vi "Word_Format_Table_Range.vi"(4 "end column":i32, 5 "start column":i32, 6 "end row":i32, 7 "start row":i32, 8 "error in":errorcluster, 9 "font":T1 {"font size" format="%.2f"; "strike through" items=["Unchanged", "Yes", "No"]; "underline" items=["Unchanged", "Yes", "No"]; "italic" items=["Unchanged", "Yes", "No"]; "bold" items=["Unchanged", "Yes", "No"]}, 10 "table":refnum<k7>, 11 "Word._Application":refnum<k7>) -> (0 "error out":errorcluster)   [LabVIEW 2020, in "NI_ReportGenerationToolkit.lvlib"]
uses:
  <vilib>/addons/_office/NI_ReportGenerationToolkit.lvlib
  <vilib>/addons/_office/_exclsub.llb/font.ctl
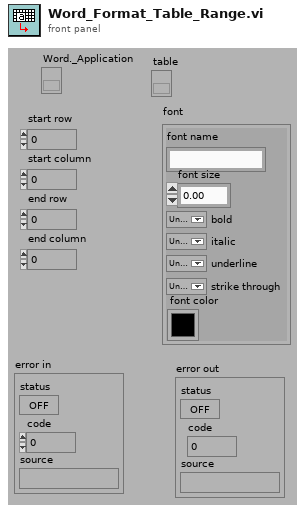
[diagram p1: front panel]
types:
  T1 = typedef "NI_ReportGenerationToolkit.lvlib/font.ctl" = cluster{"font name":string, "font size":dbl, "bold":u16, "italic":u16, "underline":u16, "strike through":u16, "font color":u32}
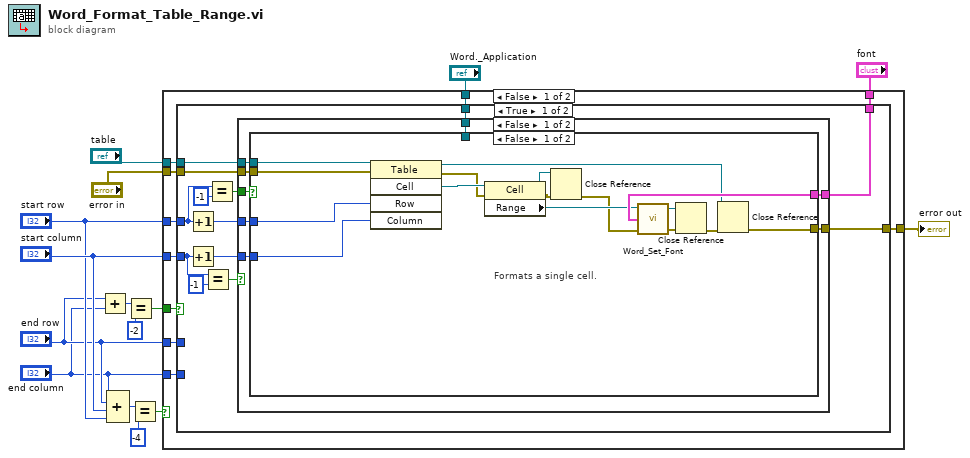
[diagram p0: block diagram]
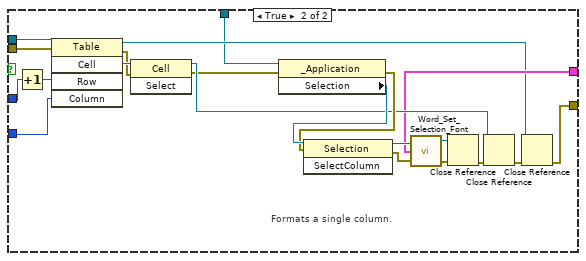
[diagram p2: hidden frame]
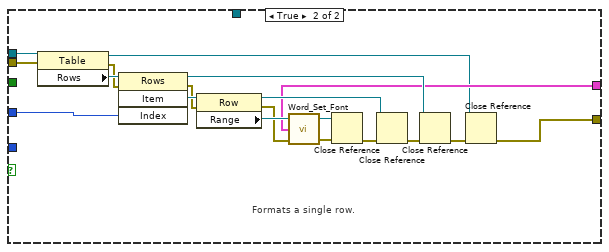
[diagram p3: hidden frame]
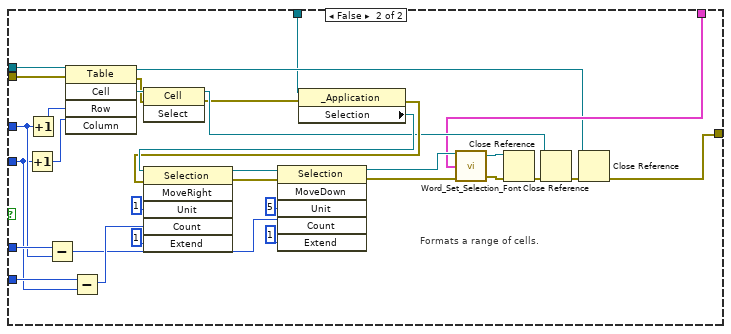
[diagram p4: hidden frame]
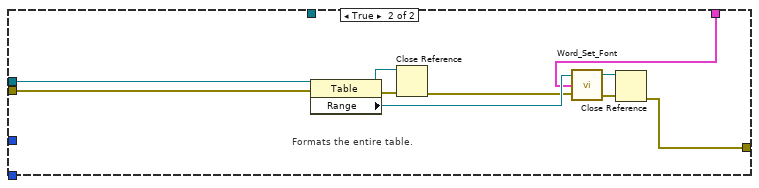
[diagram p5: hidden frame]
diagram:
  n1 = Add(x="end row", y="end column") -> (x+y=w6:i32)
  n2 = Compound Arithmetic op=ADD("end column", "end row", "start column", "start row") -> (w13:i32)
  n3 = Equal?(x=w6, y=-2) -> (x = y?=w4:bool)
  n4 = Equal?(x=w13, y=-4) -> (x = y?=w11:bool)
  n5 = case shown="False" w11 {
    tunnel: "start column" -> [w25 _]
    tunnel: "start row" -> [w24 _]
    tunnel: "end row" -> [w23 _]
    tunnel: "end column" -> [w22 _]
    tunnel: [w21 w138] -> w3
    tunnel: "table" -> [w20 w144]
    tunnel: "error in" -> [w19 w143]
    tunnel: w4 -> [w18 _]
    tunnel: "font" -> [w17 w141]
    tunnel: "Word._Application" -> [w16 _]
    frame False {
      n6 = case shown="True" w18 {
        tunnel: w25 -> [w31 w117]
        tunnel: w24 -> [w28 w118]
        tunnel: w23 -> [_ w120]
        tunnel: w22 -> [_ w119]
        tunnel: [w38 w107] -> w21
        tunnel: w20 -> [w36 w134]
        tunnel: w19 -> [w33 w133]
        tunnel: w17 -> [w37 w106]
        tunnel: w16 -> [w26 w103]
        frame True {
          n7 = Increment(x=w28) -> (x+1=w35:i32)
          n8 = Increment(x=w31) -> (x+1=w34:i32)
          n9 = Equal?(x=w31, y=-1) -> (x = y?=w32:bool)
          n10 = Equal?(x=w28, y=-1) -> (x = y?=w27:bool)
          n11 = case shown="False" w32 {
            tunnel: [w46 w85] -> w38
            tunnel: w37 -> [w45 w87]
            tunnel: w36 -> [w44 w102]
            tunnel: w35 -> [w43 w100]
            tunnel: w34 -> [w42 _]
            tunnel: w33 -> [w41 w92]
            tunnel: w27 -> [w40 _]
            tunnel: w26 -> [w39 _]
            frame False {
              n12 = case shown="False" w40 {
                tunnel: [w48 w72] -> w46
                tunnel: w45 -> [w58 w67]
                tunnel: w44 -> [w57 w81]
                tunnel: w43 -> [w56 w79]
                tunnel: w42 -> [w55 w78]
                tunnel: w41 -> [w53 w80]
                tunnel: w39 -> [_ w63]
                frame False {
                  # "Formats a single cell."
                  n13 = invoke class="Table" method="Cell"(reference=w57, error in=w53, "Row"=w56, "Column"=w55) -> (reference out=w47:refnum<k7>, error out=w52:errorcluster, "Cell"=w54:refnum<k7>)  [unwired: 1 in, 2 out]
                  n14 = property class="Cell"(reference=w54, error in=w52) -> (reference out=w62:refnum<k7>, error out=w61:errorcluster, "Range"=w51:refnum<k7>)
                  n15 = Close Reference(reference=w62, error in (no error)=w61) -> (error out=w50:errorcluster)
                  n16 = call <vilib>:"Word_Set_Font.vi"("Range in"=w51, "font"=w58, "Error in"=w50) -> ("Range out"=w59:refnum<k7>, "Error out"=w60:errorcluster)  [unwired: 5 out]
                  n17 = Close Reference(reference=w59, error in (no error)=w60) -> (error out=w49:errorcluster)
                  n18 = Close Reference(reference=w47, error in (no error)=w49) -> (error out=w48:errorcluster)
                }
                frame True {
                  # "Formats a single column."
                  n19 = Increment(x=w79) -> (x+1=w66:i32)
                  n20 = invoke class="Table" method="Cell"(reference=w81, error in=w80, "Row"=w66, "Column"=w78) -> (reference out=w65:refnum<k7>, error out=w76:errorcluster, "Cell"=w77:refnum<k7>)  [unwired: 1 in, 2 out]
                  n21 = invoke class="Cell" method="Select"(reference=w77, error in=w76) -> (reference out=w68:refnum<k7>, error out=w64:errorcluster)  [unwired: 1 in, 1 out]
                  n22 = property class="_Application"(reference=w63, error in=w64) -> (error out=w70:errorcluster, "Selection"=w71:refnum<k7>)  [unwired: 1 out]
                  n23 = invoke class="Selection" method="SelectColumn"(reference=w71, error in=w70) -> (reference out=w74:refnum<k7>, error out=w69:errorcluster)  [unwired: 1 in, 1 out]
                  n24 = call <vilib>:"Word_Set_Selection_Font.vi"("selection in"=w74, "font"=w67, "error in"=w69) -> ("selection out"=w75:refnum<k7>, "error out"=w83:errorcluster)  [unwired: 5 out]
                  n25 = Close Reference(reference=w75, error in (no error)=w83) -> (error out=w82:errorcluster)
                  n26 = Close Reference(reference=w68, error in (no error)=w82) -> (error out=w73:errorcluster)
                  n27 = Close Reference(reference=w65, error in (no error)=w73) -> (error out=w72:errorcluster)
                }
              }
            }
            frame True {
              # "Formats a single row."
              n28 = property class="Table"(reference=w102, error in=w92) -> (reference out=w84:refnum<k7>, error out=w95:errorcluster, "Rows"=w101:refnum<k7>)
              n29 = invoke class="Rows" method="Item"(reference=w101, error in=w95, "Index"=w100) -> (reference out=w88:refnum<k7>, error out=w94:errorcluster, "Item"=w99:refnum<k7>)  [unwired: 1 in, 1 out]
              n30 = property class="Row"(reference=w99, error in=w94) -> (reference out=w89:refnum<k7>, error out=w93:errorcluster, "Range"=w96:refnum<k7>)
              n31 = call <vilib>:"Word_Set_Font.vi"("Range in"=w96, "font"=w87, "Error in"=w93) -> ("Range out"=w97:refnum<k7>, "Error out"=w98:errorcluster)  [unwired: 5 out]
              n32 = Close Reference(reference=w97, error in (no error)=w98) -> (error out=w91:errorcluster)
              n33 = Close Reference(reference=w89, error in (no error)=w91) -> (error out=w90:errorcluster)
              n34 = Close Reference(reference=w88, error in (no error)=w90) -> (error out=w86:errorcluster)
              n35 = Close Reference(reference=w84, error in (no error)=w86) -> (error out=w85:errorcluster)
            }
          }
        }
        frame False {
          # "Formats a range of cells."
          n36 = Increment(x=w117) -> (x+1=w131:i32)
          n37 = Increment(x=w118) -> (x+1=w132:i32)
          n38 = Subtract(x=w120, y=w118) -> (x-y=w115:i32)
          n39 = invoke class="Table" method="Cell"(reference=w134, error in=w133, "Row"=w132, "Column"=w131) -> (reference out=w105:refnum<k7>, error out=w129:errorcluster, "Cell"=w130:refnum<k7>)  [unwired: 1 in, 2 out]
          n40 = Subtract(x=w119, y=w117) -> (x-y=w116:i32)
          n41 = invoke class="Cell" method="Select"(reference=w130, error in=w129) -> (reference out=w108:refnum<k7>, error out=w104:errorcluster)  [unwired: 1 in, 1 out]
          n42 = property class="_Application"(reference=w103, error in=w104) -> (error out=w127:errorcluster, "Selection"=w128:refnum<k7>)  [unwired: 1 out]
          n43 = invoke class="Selection" method="MoveRight"(reference=w128, error in=w127, "Unit"=1, "Count"=w116, "Extend"=1) -> (reference out=w124:refnum<k7>, error out=w123:errorcluster)  [unwired: 1 in, 4 out]
          n44 = invoke class="Selection" method="MoveDown"(reference=w124, error in=w123, "Unit"=5, "Count"=w115, "Extend"=1) -> (reference out=w113:refnum<k7>, error out=w114:errorcluster)  [unwired: 1 in, 4 out]
          n45 = call <vilib>:"Word_Set_Selection_Font.vi"("selection in"=w113, "font"=w106, "error in"=w114) -> ("selection out"=w109:refnum<k7>, "error out"=w110:errorcluster)  [unwired: 5 out]
          n46 = Close Reference(reference=w109, error in (no error)=w110) -> (error out=w112:errorcluster)
          n47 = Close Reference(reference=w108, error in (no error)=w112) -> (error out=w111:errorcluster)
          n48 = Close Reference(reference=w105, error in (no error)=w111) -> (error out=w107:errorcluster)
        }
      }
    }
    frame True {
      # "Formats the entire table."
      n49 = property class="Table"(reference=w144, error in=w143) -> (reference out=w135:refnum<k7>, error out=w137:errorcluster, "Range"=w142:refnum<k7>)
      n50 = Close Reference(reference=w135, error in (no error)=w137) -> (error out=w136:errorcluster)
      n51 = call <vilib>:"Word_Set_Font.vi"("Range in"=w142, "font"=w141, "Error in"=w136) -> ("Range out"=w139:refnum<k7>, "Error out"=w140:errorcluster)  [unwired: 5 out]
      n52 = Close Reference(reference=w139, error in (no error)=w140) -> (error out=w138:errorcluster)
    }
  }
  "error out" <- w3
